vi "Identify.vi"(8 "error in (no error)":errorcluster, 11 "Skyworks - 2G PVT in":refnum<class "Skyworks - PA Modeswitch.lvclass">) -> (0 "error out":errorcluster, 2 "Plugin is Valid":bool, 3 "Skyworks - 2G PVT out":refnum<class "Skyworks - PA Modeswitch.lvclass">)   [LabVIEW 2016, in "Skyworks - PA Modeswitch.lvlib" / "Skyworks - PA Modeswitch.lvclass"]
uses:
  Skyworks - PA Modeswitch.lvclass
  C:/Sequence Automation/Plugins/Measurement Interface.lvlibp/Measurement Interface.lvclass
  C:/Sequence Automation/Plugins/Measurements/Skyworks - PVT.lvlibp/Skyworks - PVT.lvclass
  Plugins/Measurement Interface.lvlibp/Private Methods/Measurement Definition Entry/Read Measurement Definition Entry.vi
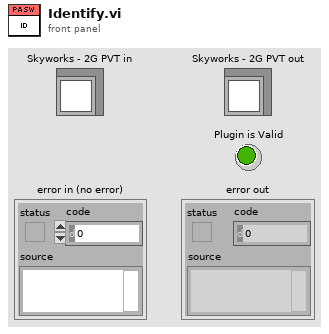
[diagram p1: front panel]
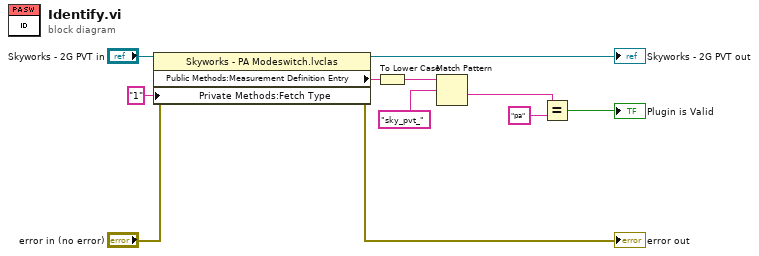
[diagram p0: block diagram]
diagram:
  n1 = property class="Skyworks - PA Modeswitch.lvclas"(reference="Skyworks - 2G PVT in", error in="error in (no error)", "Private Methods:Fetch Type"="1" ("Fetch Type")) -> (reference out=→"Skyworks - 2G PVT out":refnum<class "Skyworks - PA Modeswitch.lvclass">, error out=→"error out":errorcluster, "Public Methods:Measurement Definition Entry"=w11:string)
  n2 = To Lower Case(string=w11) -> (all lower case string=w9:string)
  n3 = Match Pattern(string=w9, regular expression="sky_pvt_") -> (after substring=w8:string)  [unwired: 1 in, 3 out]
  n4 = Equal?(x=w8, y="pa") -> (x = y?=→"Plugin is Valid":bool)
